vi "Run Config Data Decoder.vi"(8 "error in (no error)":errorcluster, 11 "Data":variant) -> (0 "error out":errorcluster, 3 "Run Config Data":T1)   [LabVIEW 2026, in "TALOS.lvlib" / "Guardian.lvlib" / "Guardian.lvclass"]
uses:
  Guardian.lvclass
  Run Config Data.ctl
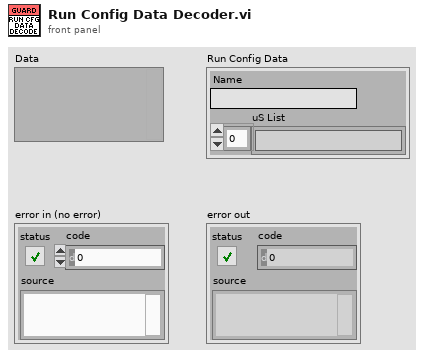
[diagram p1: front panel]
types:
  T1 = typedef "TALOS.lvlib/Guardian.lvlib/Guardian.lvclass/Run Config Data.ctl" = cluster{"Name":string, "uS List":string[]}
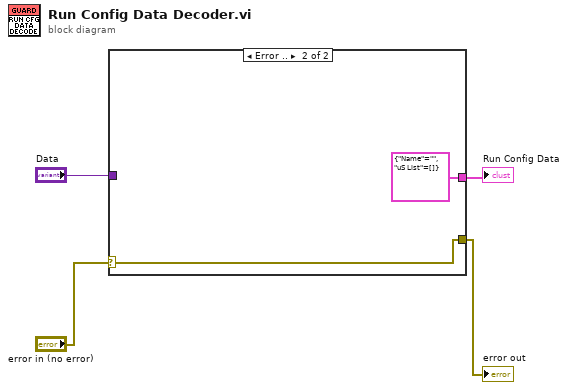
[diagram p0: block diagram]
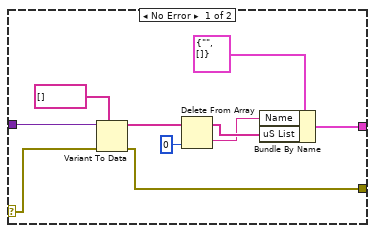
[diagram p2: hidden frame]
diagram:
  n1 = case shown="Error .." "error in (no error)" {
    selector: "error in (no error)" -> [w13 w15]
    tunnel: [w14 w15] -> w4
    tunnel: "Data" -> [w12 _]
    tunnel: [w5 T1 {"Name"="", "uS List"=[]} ("Run Config Data")] -> w1
    frame No Error {
      n2 = Variant To Data(error in=w13, type=string[] [], Variant=w12) -> (data=w10:string[], error out=w14:errorcluster)
      n3 = Delete From Array(array=w10, index=0) -> (deleted portion=w6:string, array with subset deleted=w7:string[])  [unwired: 1 in]
      n4 = Bundle By Name(cluster=T1 {"Name"="", "uS List"=[]} ("Run Config Data"), "Name"=w6, "uS List"=w7) -> (w5:T1)
    }
    frame Error {
    }
  }
  "Run Config Data" <- w1
  "error out" <- w4
